vi "DataCANFileInfo.vi"(9 "Language":u32, 11 "file path (dialog if empty)":path caption="文件路径 （空时为对话框）") -> (0 "路径输出":path, 2 "FileInfo":string, 3 "文件类型":string)   [LabVIEW 2015]
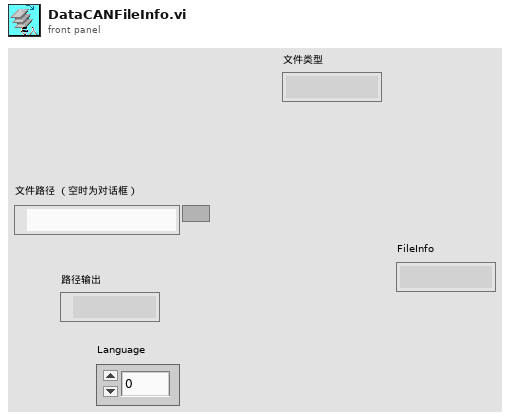
[diagram p1: front panel]
types:
  T1 = enum16{"open", "replace", "create", "open or create", "replace or create", "replace or create with confirmation"}
  T2 = enum16{"big-endian, network order", "native, host order", "little-endian"}
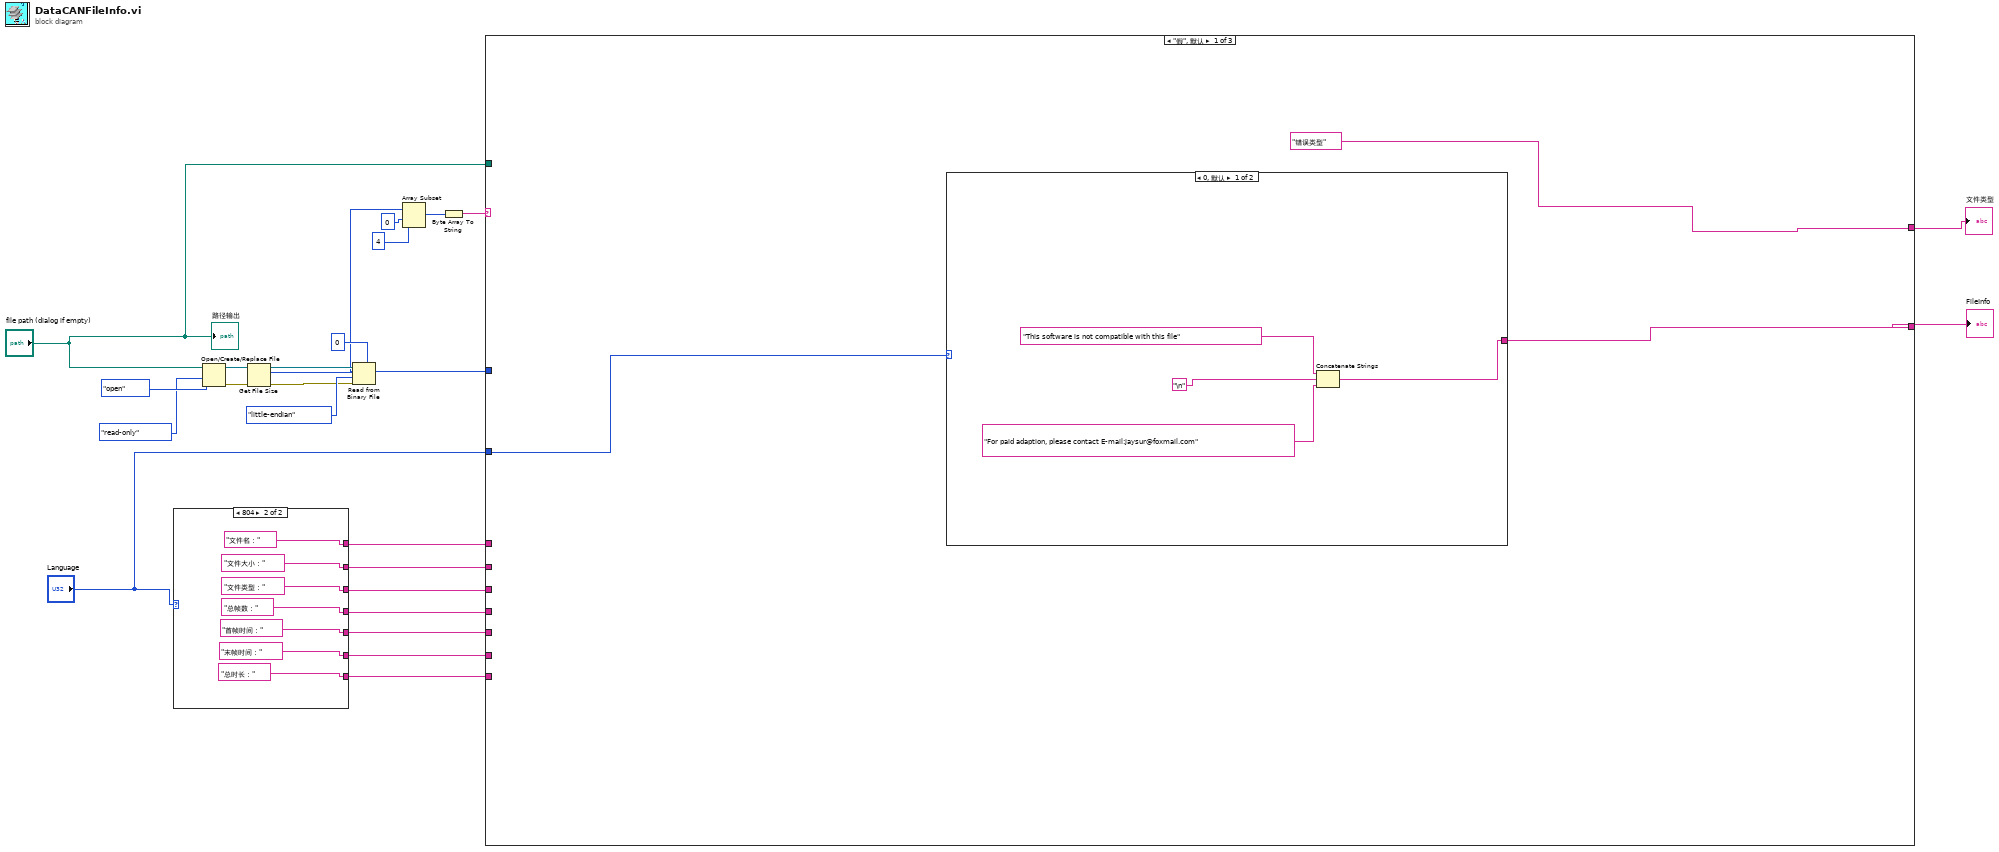
[diagram p0: block diagram]
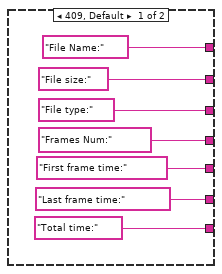
[diagram p2: hidden frame]
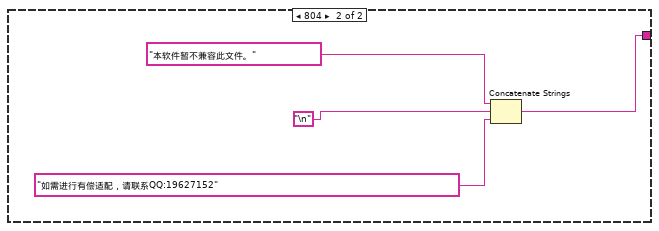
[diagram p3: hidden frame]
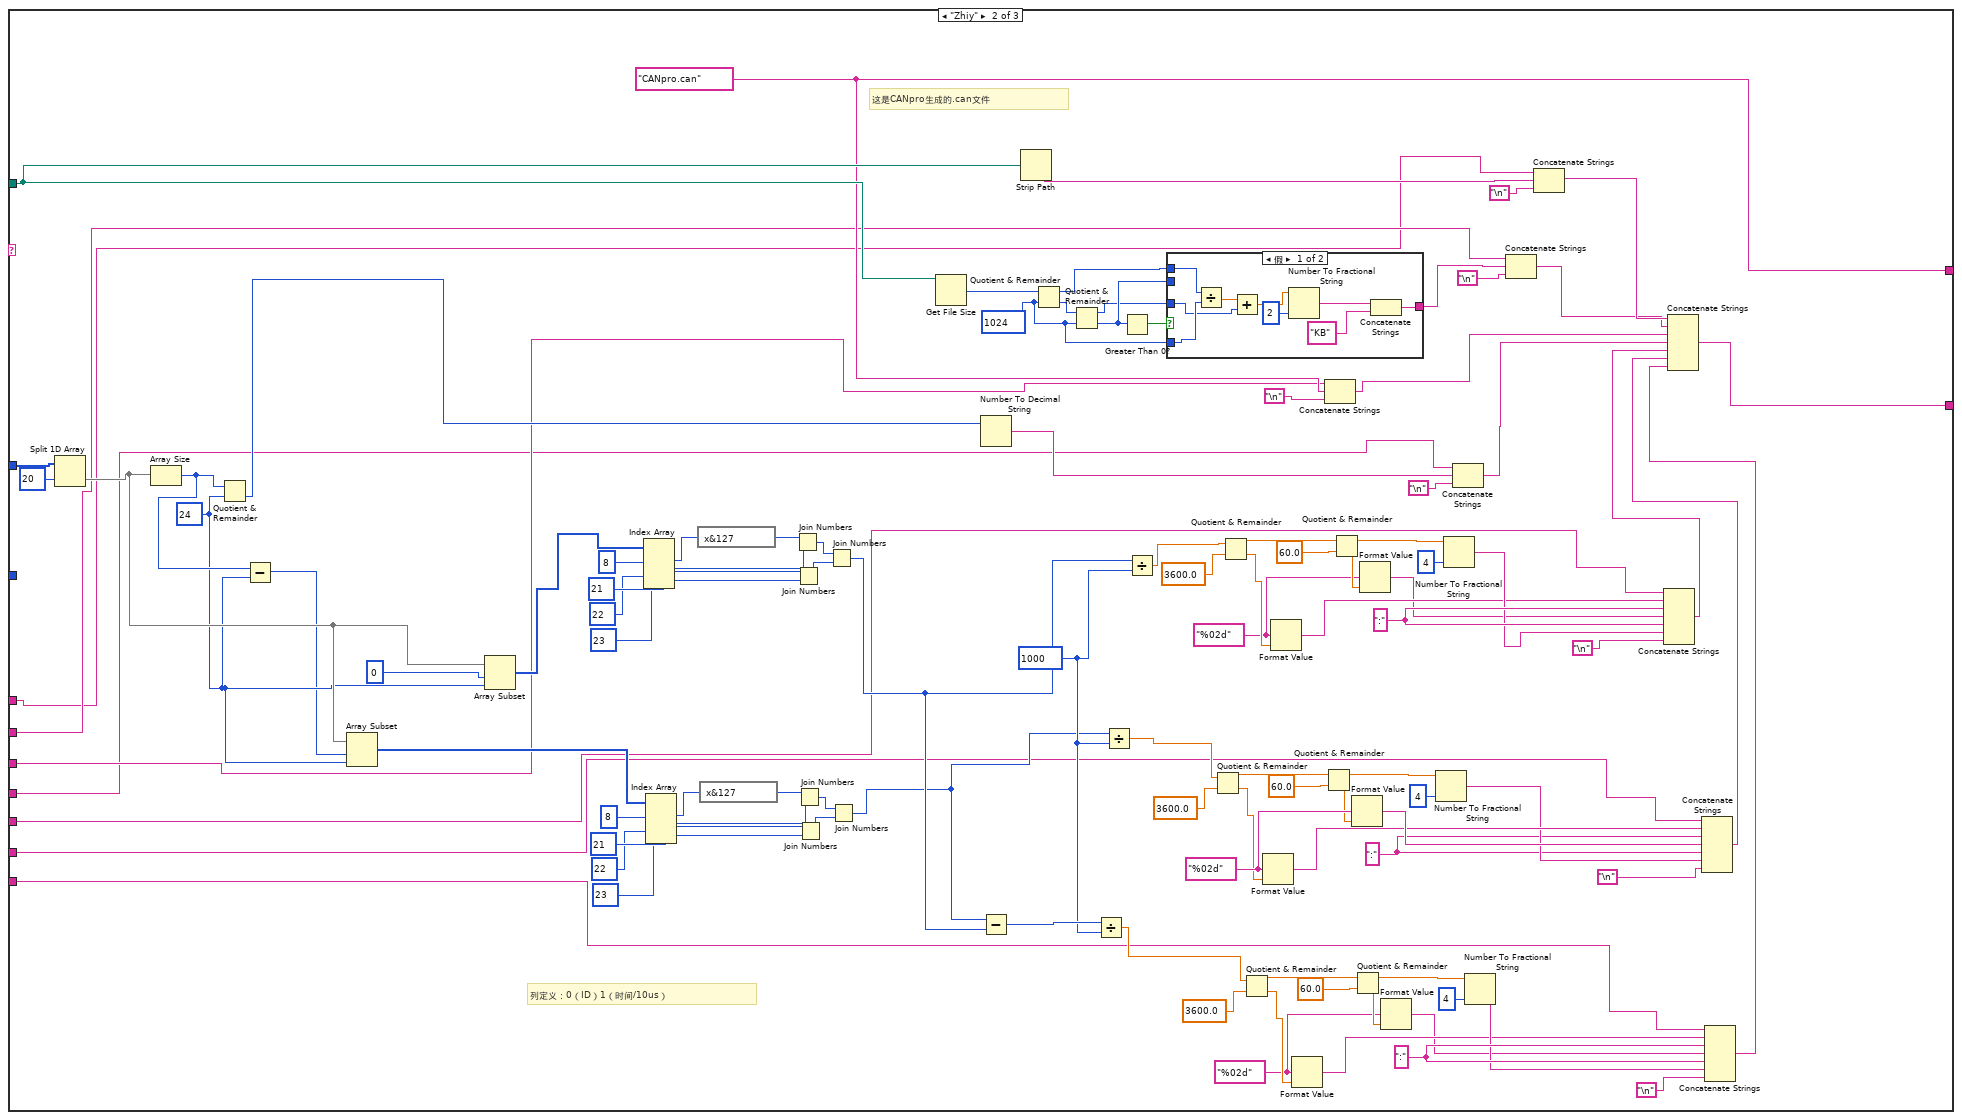
[diagram p4: hidden frame]
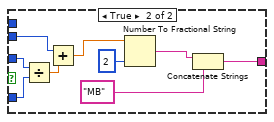
[diagram p5: hidden frame]
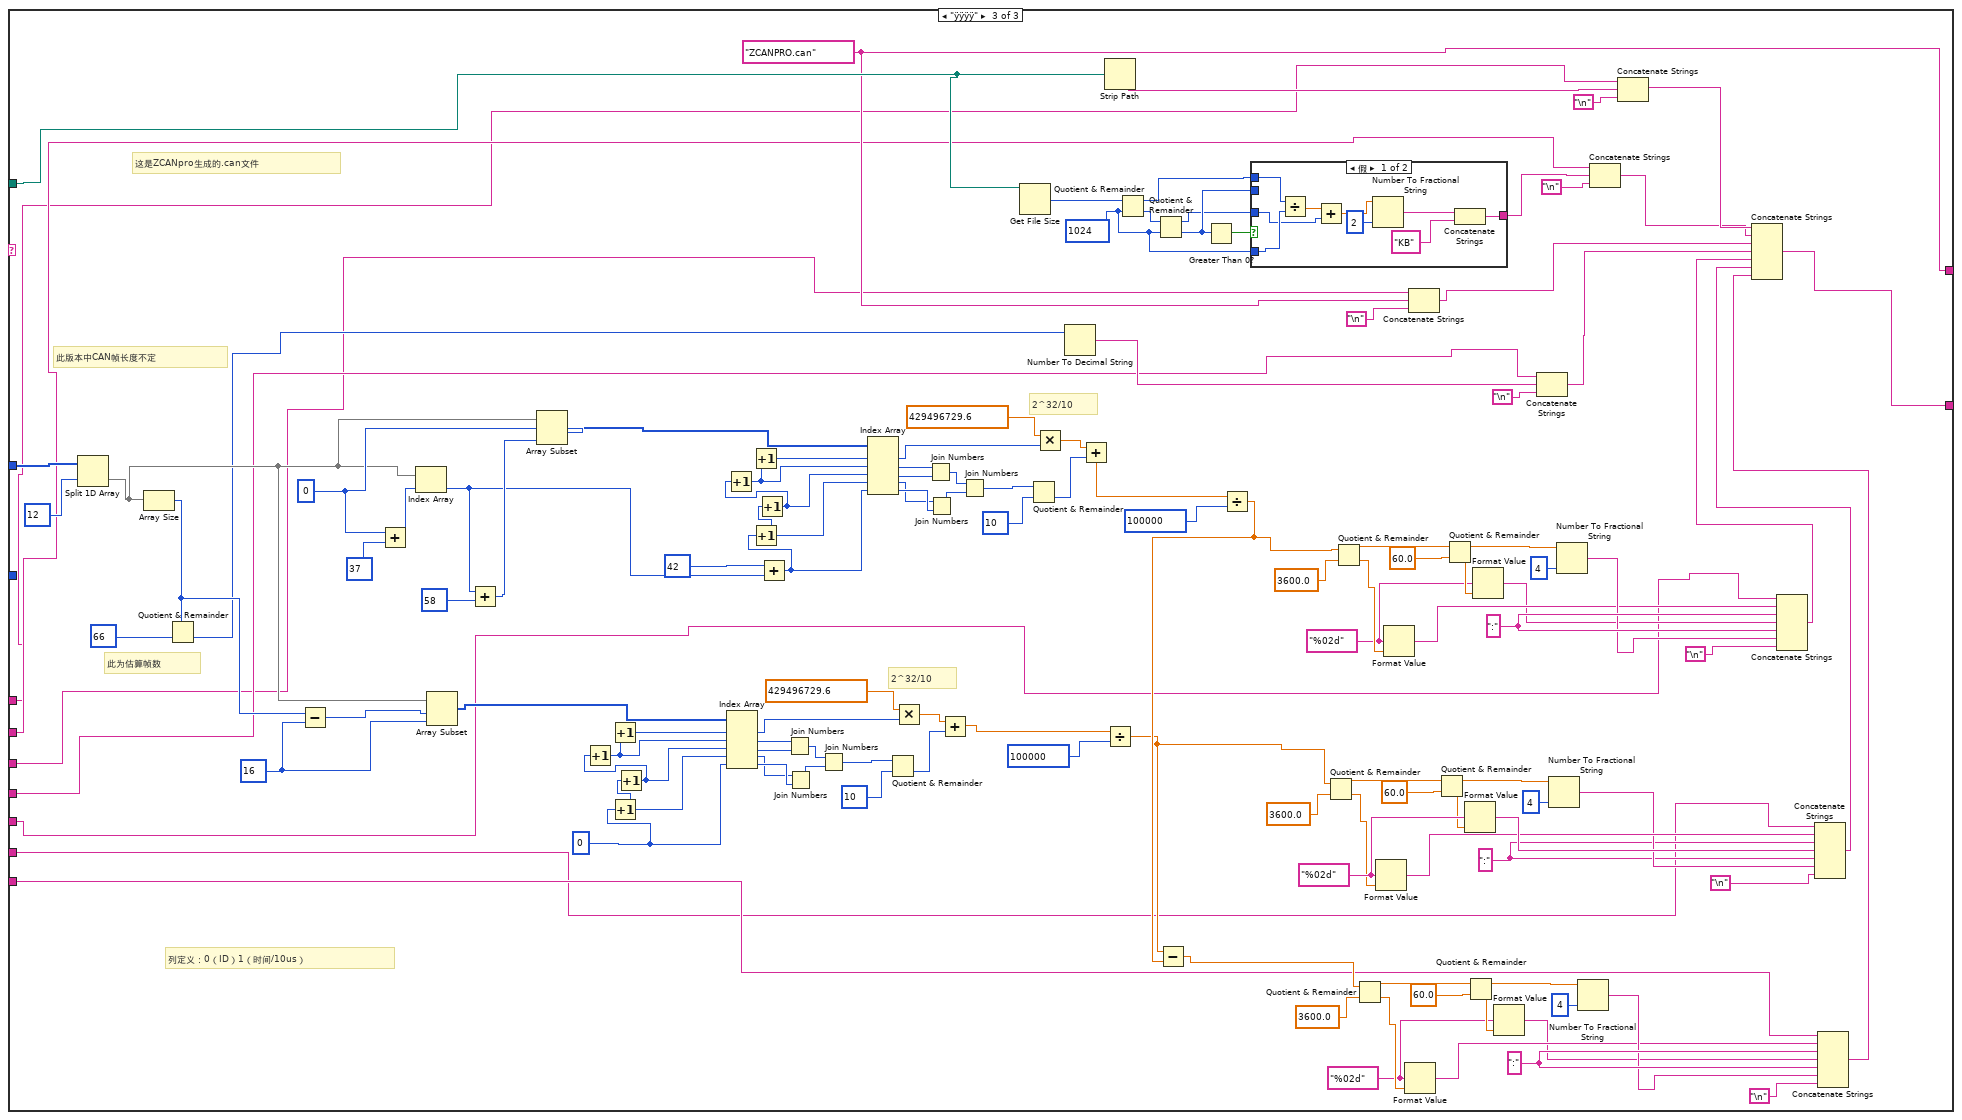
[diagram p6: hidden frame]
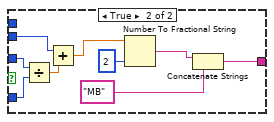
[diagram p7: hidden frame]
diagram:
  n1 = case shown="804" "Language" {
    tunnel: ["Total time:" "总时长："] -> w2
    tunnel: ["Last frame time:" "末帧时间："] -> w3
    tunnel: ["First frame time:" "首帧时间："] -> w4
    tunnel: ["Frames Num:" "总帧数："] -> w5
    tunnel: ["File type:" "文件类型："] -> w6
    tunnel: ["File size:" "文件大小："] -> w7
    tunnel: ["File Name:" "文件名："] -> w8
    frame 409, Default {
    }
    frame 804 {
    }
  }
  n2 = Open/Create/Replace File(file path (use dialog)="file path (dialog if empty)", operation (0:open)=T1."open" ("操作(0:open)"), access (0:read/write)=enum16{"read/write", "read-only", "write-only"}."read-only" ("权限(0:read/write)")) -> (refnum out=w17:refnum<file>, error out=w22:errorcluster)  [unwired: 3 in, 1 out]
  n3 = Get File Size(file=w17, error in=w22) -> (refnum out=w20:refnum<file>, size (in bytes)=w21:i64, 0:w19:errorcluster)
  n4 = Read from Binary File(5:u8 0, 8:w19, 9:T2."little-endian" ("字节顺序(0:big-endian, network order)"), 10:w21, 11:w20) -> (2:w13:u8[])  [unwired: 1 in, 3 out]
  n5 = Array Subset(array=w13, index=0 ("索引"), length=4 ("长度")) -> (w14:u8[])
  n6 = Byte Array To String(unsigned byte array=w14) -> (string=w12:string)
  n7 = case shown="\"假\", 默认" w12 {
    tunnel: w13 -> [_ w158 w304]
    tunnel: "file path (dialog if empty)" -> [_ w90 w191]
    tunnel: [w42 w91 w192] -> w10
    tunnel: ["错误类型" w58 w185] -> w9
    tunnel: w8 -> [_ w55 w178]
    tunnel: w7 -> [_ w56 w179]
    tunnel: w6 -> [_ w57 w180]
    tunnel: w5 -> [_ w51 w181]
    tunnel: w4 -> [_ w52 w182]
    tunnel: w3 -> [_ w53 w183]
    tunnel: w2 -> [_ w54 w184]
    tunnel: "Language" -> [w41 _ _]
    frame "假", Default {
      n8 = case shown="0, 默认" w41 {
        tunnel: [w43 w47] -> w42
        frame 0, Default {
          n9 = Concatenate Strings("This software is not compatible with this file", "\n", "For paid adaption, please contact E-mail:jaysur@foxmail.com") -> (w43:string)
        }
        frame 804 {
          n10 = Concatenate Strings("本软件暂不兼容此文件。", "\n", "如需进行有偿适配，请联系QQ:19627152") -> (w47:string)
        }
      }
    }
    frame "Zhiy" {
      w96 = i64 1024 ("y")
      w116 = "%02d" ("格式字符串")
      w122 = ":"
      w139 = "%02d" ("格式字符串")
      w133 = ":"
      w140 = "%02d" ("格式字符串")
      w146 = ":"
      w58 = "CANpro.can"
      w73 = u32 1000 ("y")
      w154 = 24 ("y")
      # "列定义：0（ID）1（时间/10us）"
      # "这是CANpro生成的.can文件"
      n11 = Split 1D Array(array=w158, index=20 ("索引")) -> (second subarray=w156:u8[])  [unwired: 1 out]
      n12 = Array Size(array=w156) -> (size(s)=w155:i32)
      n13 = Quotient & Remainder(x=w155, y=w154) -> (floor(x/y)=w89:i32)  [unwired: 1 out]
      n14 = Subtract(x=w155, y=w154) -> (x-y=w153:i32)
      n15 = Array Subset(array=w156, index=w153, length=w154) -> (w59:u8[])
      n16 = Array Subset(array=w156, index=0 ("索引"), length=w154) -> (w74:u8[])
      n17 = Index Array(array=w74, index #1=8 ("索引"), index #2=21 ("索引"), index #3=22 ("索引"), index #4=23 ("索引")) -> (element #1=w76:u8, element #2=w79:u8, element #3=w78:u8, element #4=w77:u8)
      n18 = Index Array(array=w59, index #1=8 ("索引"), index #2=21 ("索引"), index #3=22 ("索引"), index #4=23 ("索引")) -> (element #1=w62:u8, element #2=w65:u8, element #3=w64:u8, element #4=w63:u8)
      n19 = expression code="x&127"(w76) -> (w75:u8)
      n20 = expression code="x&127"(w62) -> (w61:u8)
      n21 = Join Numbers(hi=w75, lo=w79) -> ((hi.lo)=w80:u16)
      n22 = Join Numbers(hi=w78, lo=w77) -> ((hi.lo)=w81:u16)
      n23 = Join Numbers(hi=w61, lo=w65) -> ((hi.lo)=w66:u16)
      n24 = Join Numbers(hi=w64, lo=w63) -> ((hi.lo)=w67:u16)
      n25 = Join Numbers(hi=w80, lo=w81) -> ((hi.lo)=w72:u32)
      n26 = Join Numbers(hi=w66, lo=w67) -> ((hi.lo)=w60:u32)
      n27 = Get File Size(file=w90) -> (size (in bytes)=w99:i64)  [unwired: 1 in, 2 out]
      n28 = Number To Decimal String(number=w89) -> (decimal integer string=w102:string)  [unwired: 1 in]
      n29 = Subtract(x=w60, y=w72) -> (x-y=w152:u32)
      n30 = Strip Path(path=w90) -> (name=w109:string)  [unwired: 1 out]
      n31 = Quotient & Remainder(x=w99, y=w96) -> (x-y*floor(x/y)=w92:i64, floor(x/y)=w98:i64)
      n32 = Quotient & Remainder(x=w98, y=w96) -> (x-y*floor(x/y)=w94:i64, floor(x/y)=w95:i64)
      n33 = Divide(x=w152, y=w73) -> (x/y=w112:dbl)
      n34 = Divide(x=w60, y=w73) -> (x/y=w111:dbl)
      n35 = Greater Than 0?(x=w95) -> (x > 0?=w97:bool)
      n36 = Divide(x=w72, y=w73) -> (x/y=w110:dbl)
      n37 = case shown="假" w97 {
        tunnel: w96 -> [w165 w175]
        tunnel: w95 -> [_ w173]
        tunnel: w94 -> [w163 w176]
        tunnel: [w168 w171] -> w93
        tunnel: w92 -> [w166 _]
        frame False {
          n38 = Divide(x=w166, y=w165) -> (x/y=w164:dbl)
          n39 = Add(x=w164, y=w163) -> (x+y=w162:dbl)
          n40 = Number To Fractional String(number=w162, precision (6)=i16 2 ("精度(6)")) -> (F-format string=w160:string)  [unwired: 2 in]
          n41 = Concatenate Strings(w160, "KB" ("字符串")) -> (w168:string)
        }
        frame True {
          n42 = Divide(x=w176, y=w175) -> (x/y=w174:dbl)
          n43 = Add(x=w173, y=w174) -> (x+y=w172:dbl)
          n44 = Number To Fractional String(number=w172, precision (6)=i16 2 ("精度(6)")) -> (F-format string=w170:string)  [unwired: 2 in]
          n45 = Concatenate Strings(w170, "MB") -> (w171:string)
        }
      }
      n46 = Quotient & Remainder(x=w111, y=3600.0) -> (x-y*floor(x/y)=w129:dbl, floor(x/y)=w136:dbl)
      n47 = Quotient & Remainder(x=w110, y=3600.0) -> (x-y*floor(x/y)=w150:dbl, floor(x/y)=w143:dbl)
      n48 = Quotient & Remainder(x=w112, y=3600.0) -> (x-y*floor(x/y)=w126:dbl, floor(x/y)=w119:dbl)
      n49 = Format Value(format string=w139, value (0)=w136) -> (output string=w135:string)  [unwired: 1 in]
      n50 = Format Value(format string=w140, value (0)=w143) -> (output string=w144:string)  [unwired: 1 in]
      n51 = Format Value(format string=w116, value (0)=w119) -> (output string=w120:string)  [unwired: 1 in]
      n52 = Quotient & Remainder(x=w129, y=60.0) -> (x-y*floor(x/y)=w131:dbl, floor(x/y)=w137:dbl)
      n53 = Concatenate Strings(w57, w58, "\n") -> (w106:string)
      n54 = Quotient & Remainder(x=w150, y=60.0) -> (x-y*floor(x/y)=w148:dbl, floor(x/y)=w142:dbl)
      n55 = Format Value(format string=w139, value (0)=w137) -> (output string=w138:string)  [unwired: 1 in]
      n56 = Quotient & Remainder(x=w126, y=60.0) -> (x-y*floor(x/y)=w124:dbl, floor(x/y)=w118:dbl)
      n57 = Format Value(format string=w140, value (0)=w142) -> (output string=w141:string)  [unwired: 1 in]
      n58 = Format Value(format string=w116, value (0)=w118) -> (output string=w117:string)  [unwired: 1 in]
      n59 = Number To Fractional String(number=w131, precision (6)=i16 4 ("精度(6)")) -> (F-format string=w134:string)  [unwired: 2 in]
      n60 = Number To Fractional String(number=w148, precision (6)=i16 4 ("精度(6)")) -> (F-format string=w145:string)  [unwired: 2 in]
      n61 = Concatenate Strings(w51, w102, "\n") -> (w103:string)
      n62 = Number To Fractional String(number=w124, precision (6)=i16 4 ("精度(6)")) -> (F-format string=w121:string)  [unwired: 2 in]
      n63 = Concatenate Strings(w56, w93, "\n") -> (w100:string)
      n64 = Concatenate Strings(w55, w109, "\n") -> (w108:string)
      n65 = Concatenate Strings(w52, w144, w146, w141, w146, w145, "\n") -> (w88:string)
      n66 = Concatenate Strings(w53, w135, w133, w138, w133, w134, "\n") -> (w87:string)
      n67 = Concatenate Strings(w54, w120, w122, w117, w122, w121, "\n") -> (w86:string)
      n68 = Concatenate Strings(w108, w100, w106, w103, w88, w87, w86) -> (w91:string)
    }
    frame "ÿÿÿÿ" {
      w197 = i64 1024 ("y")
      w216 = "%02d" ("格式字符串")
      w222 = ":"
      w239 = "%02d" ("格式字符串")
      w233 = ":"
      w240 = "%02d" ("格式字符串")
      w246 = ":"
      w185 = "ZCANPRO.can"
      w257 = 0 ("x+y")
      w276 = 16 ("长度")
      w302 = 0
      # "2^32/10"
      # "2^32/10"
      # "列定义：0（ID）1（时间/10us）"
      # "此为估算帧数"
      # "此版本中CAN帧长度不定"
      # "这是ZCANpro生成的.can文件"
      n69 = Split 1D Array(array=w304, index=12 ("索引")) -> (second subarray=w277:u8[])  [unwired: 1 out]
      n70 = Array Size(array=w277) -> (size(s)=w275:i32)
      n71 = Quotient & Remainder(x=w275, y=66) -> (floor(x/y)=w190:i32)  [unwired: 1 out]
      n72 = Subtract(x=w275, y=w276) -> (x-y=w252:i32)
      n73 = Add(x=w302, y=37) -> (x+y=w288:i32)
      n74 = Index Array(array=w277, index=w288) -> (element=w278:u8)
      n75 = Array Subset(array=w277, index=w252, length=w276) -> (w258:u8[])
      n76 = Add(x=w278, y=u8 58) -> (x+y=w285:u8)
      n77 = Array Subset(array=w277, index=w302, length=w285) -> (w295:u8[])
      n78 = Increment(x=w257) -> (x+1=w262:i32)
      n79 = Increment(x=w262) -> (x+1=w261:i32)
      n80 = Increment(x=w261) -> (x+1=w259:i32)
      n81 = Increment(x=w259) -> (x+1=w260:i32)
      n82 = Index Array(array=w258, index #1=w260, index #2=w259, index #3=w261, index #4=w262, index #5=w257) -> (element #1=w266:u8, element #2=w269:u8, element #3=w270:u8, element #4=w271:u8, element #5=w272:u8)
      n83 = Add(x=42 ("索引"), y=w278) -> (x+y=w283:i32)
      n84 = Increment(x=w283) -> (x+1=w282:i32)
      n85 = Increment(x=w282) -> (x+1=w281:i32)
      n86 = Increment(x=w281) -> (x+1=w279:i32)
      n87 = Increment(x=w279) -> (x+1=w280:i32)
      n88 = Join Numbers(hi=w269, lo=w270) -> ((hi.lo)=w273:u16)
      n89 = Join Numbers(hi=w271, lo=w272) -> ((hi.lo)=w274:u16)
      n90 = Join Numbers(hi=w273, lo=w274) -> ((hi.lo)=w268:u32)
      n91 = Index Array(array=w295, index #1=w280, index #2=w279, index #3=w281, index #4=w282, index #5=w283) -> (element #1=w292:u8, element #2=w296:u8, element #3=w297:u8, element #4=w298:u8, element #5=w299:u8)
      n92 = Quotient & Remainder(x=w268, y=u32 10) -> (floor(x/y)=w263:u32)  [unwired: 1 out]
      n93 = Multiply(x=429496729.6, y=w266) -> (x*y=w264:dbl)
      n94 = Join Numbers(hi=w296, lo=w297) -> ((hi.lo)=w300:u16)
      n95 = Join Numbers(hi=w298, lo=w299) -> ((hi.lo)=w301:u16)
      n96 = Add(x=w264, y=w263) -> (x+y=w254:dbl)
      n97 = Join Numbers(hi=w300, lo=w301) -> ((hi.lo)=w294:u32)
      n98 = Get File Size(file=w191) -> (size (in bytes)=w200:i64)  [unwired: 1 in, 2 out]
      n99 = Quotient & Remainder(x=w294, y=u32 10) -> (floor(x/y)=w289:u32)  [unwired: 1 out]
      n100 = Multiply(x=429496729.6, y=w292) -> (x*y=w290:dbl)
      n101 = Number To Decimal String(number=w190) -> (decimal integer string=w203:string)  [unwired: 1 in]
      n102 = Add(x=w290, y=w289) -> (x+y=w253:dbl)
      n103 = Strip Path(path=w191) -> (name=w209:string)  [unwired: 1 out]
      n104 = Divide(x=w254, y=i64 100000) -> (x/y=w212:dbl)
      n105 = Quotient & Remainder(x=w200, y=w197) -> (x-y*floor(x/y)=w193:i64, floor(x/y)=w199:i64)
      n106 = Quotient & Remainder(x=w199, y=w197) -> (x-y*floor(x/y)=w195:i64, floor(x/y)=w196:i64)
      n107 = Greater Than 0?(x=w196) -> (x > 0?=w198:bool)
      n108 = Divide(x=w253, y=i64 100000) -> (x/y=w213:dbl)
      n109 = Subtract(x=w212, y=w213) -> (x-y=w211:dbl)
      n110 = case shown="假" w198 {
        tunnel: w197 -> [w311 w321]
        tunnel: w196 -> [_ w319]
        tunnel: w195 -> [w309 w322]
        tunnel: [w314 w317] -> w194
        tunnel: w193 -> [w312 _]
        frame False {
          n111 = Divide(x=w312, y=w311) -> (x/y=w310:dbl)
          n112 = Add(x=w310, y=w309) -> (x+y=w308:dbl)
          n113 = Number To Fractional String(number=w308, precision (6)=i16 2 ("精度(6)")) -> (F-format string=w306:string)  [unwired: 2 in]
          n114 = Concatenate Strings(w306, "KB" ("字符串")) -> (w314:string)
        }
        frame True {
          n115 = Divide(x=w322, y=w321) -> (x/y=w320:dbl)
          n116 = Add(x=w319, y=w320) -> (x+y=w318:dbl)
          n117 = Number To Fractional String(number=w318, precision (6)=i16 2 ("精度(6)")) -> (F-format string=w316:string)  [unwired: 2 in]
          n118 = Concatenate Strings(w316, "MB") -> (w317:string)
        }
      }
      n119 = Quotient & Remainder(x=w212, y=3600.0) -> (x-y*floor(x/y)=w229:dbl, floor(x/y)=w236:dbl)
      n120 = Quotient & Remainder(x=w213, y=3600.0) -> (x-y*floor(x/y)=w250:dbl, floor(x/y)=w243:dbl)
      n121 = Quotient & Remainder(x=w211, y=3600.0) -> (x-y*floor(x/y)=w226:dbl, floor(x/y)=w219:dbl)
      n122 = Format Value(format string=w239, value (0)=w236) -> (output string=w235:string)  [unwired: 1 in]
      n123 = Format Value(format string=w240, value (0)=w243) -> (output string=w244:string)  [unwired: 1 in]
      n124 = Format Value(format string=w216, value (0)=w219) -> (output string=w220:string)  [unwired: 1 in]
      n125 = Concatenate Strings(w180, w185, "\n") -> (w206:string)
      n126 = Quotient & Remainder(x=w229, y=60.0) -> (x-y*floor(x/y)=w231:dbl, floor(x/y)=w237:dbl)
      n127 = Quotient & Remainder(x=w250, y=60.0) -> (x-y*floor(x/y)=w248:dbl, floor(x/y)=w242:dbl)
      n128 = Format Value(format string=w239, value (0)=w237) -> (output string=w238:string)  [unwired: 1 in]
      n129 = Quotient & Remainder(x=w226, y=60.0) -> (x-y*floor(x/y)=w224:dbl, floor(x/y)=w218:dbl)
      n130 = Format Value(format string=w240, value (0)=w242) -> (output string=w241:string)  [unwired: 1 in]
      n131 = Format Value(format string=w216, value (0)=w218) -> (output string=w217:string)  [unwired: 1 in]
      n132 = Concatenate Strings(w181, w203, "\n") -> (w204:string)
      n133 = Number To Fractional String(number=w231, precision (6)=i16 4 ("精度(6)")) -> (F-format string=w234:string)  [unwired: 2 in]
      n134 = Number To Fractional String(number=w248, precision (6)=i16 4 ("精度(6)")) -> (F-format string=w245:string)  [unwired: 2 in]
      n135 = Number To Fractional String(number=w224, precision (6)=i16 4 ("精度(6)")) -> (F-format string=w221:string)  [unwired: 2 in]
      n136 = Concatenate Strings(w179, w194, "\n") -> (w201:string)
      n137 = Concatenate Strings(w178, w209, "\n") -> (w208:string)
      n138 = Concatenate Strings(w182, w244, w246, w241, w246, w245, "\n") -> (w189:string)
      n139 = Concatenate Strings(w183, w235, w233, w238, w233, w234, "\n") -> (w188:string)
      n140 = Concatenate Strings(w184, w220, w222, w217, w222, w221, "\n") -> (w187:string)
      n141 = Concatenate Strings(w208, w201, w206, w204, w189, w188, w187) -> (w192:string)
    }
  }
  "FileInfo" <- w10
  "文件类型" <- w9
  "路径输出" <- "file path (dialog if empty)"
